vi "refMgr_Example4.vi"() -> ()   [LabVIEW 2017]
uses:
  RefManager/Typedef/RefMgr-Logic-State.ctl
  RefManager/Typedef/RefMgr-StateChangeType.ctl
  40be52e9-3771-4604-be95-a9dd39ca470b.vi
  <userlib>/_NEVSTOP/TagDB/_Support/DataAccess/data-Write.vi
  <userlib>/_NEVSTOP/TagDB/_Support/DataAccess/_NameCacher.vi
  <userlib>/_NEVSTOP/TagDB/_Support/DataAccess/_datatypeChecker.vi
  <userlib>/_NEVSTOP/TagDB/_Support/DataAccess/TagDB Ref to DVR.vi
  <vilib>/Utility/Data Type/Get Type Information.vi
  <vilib>/Utility/error.llb/Trim Whitespace.vi
  <userlib>/_NEVSTOP/TagDB/_Support/Error/_[error50000]Invalid DB REF.vi
  RefManager/TagDB RefManager.lvlib
  <userlib>/_NEVSTOP/TagDB/TagDB.lvlib
panel:
  in  "StateValue":i16
  in  "stop":bool
  in  "Boolean 6":bool
  in  "Boolean 5":bool
  in  "Boolean 4":bool
  in  "Boolean 3":bool
  in  "Boolean 2":bool
  in  "Boolean 1":bool
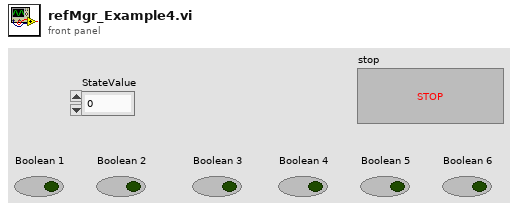
[diagram p1: front panel]
types:
  T1 = typedef "TagDB RefManager.lvlib/RefMgr-Logic-State.ctl" = cluster{"StateName":string, "StateValue":i32, "Type":T2, "Calcs":cluster{"Tag":string, "Exp":string}[]}
  T2 = typedef "TagDB RefManager.lvlib/RefMgr-StateChangeType.ctl" = enum16{"0 - 进入", "1 - 等于", "2 - 退出"}
  T3 = typedef "TagDB.lvlib/TagDB.ctl" = refnum<k1>
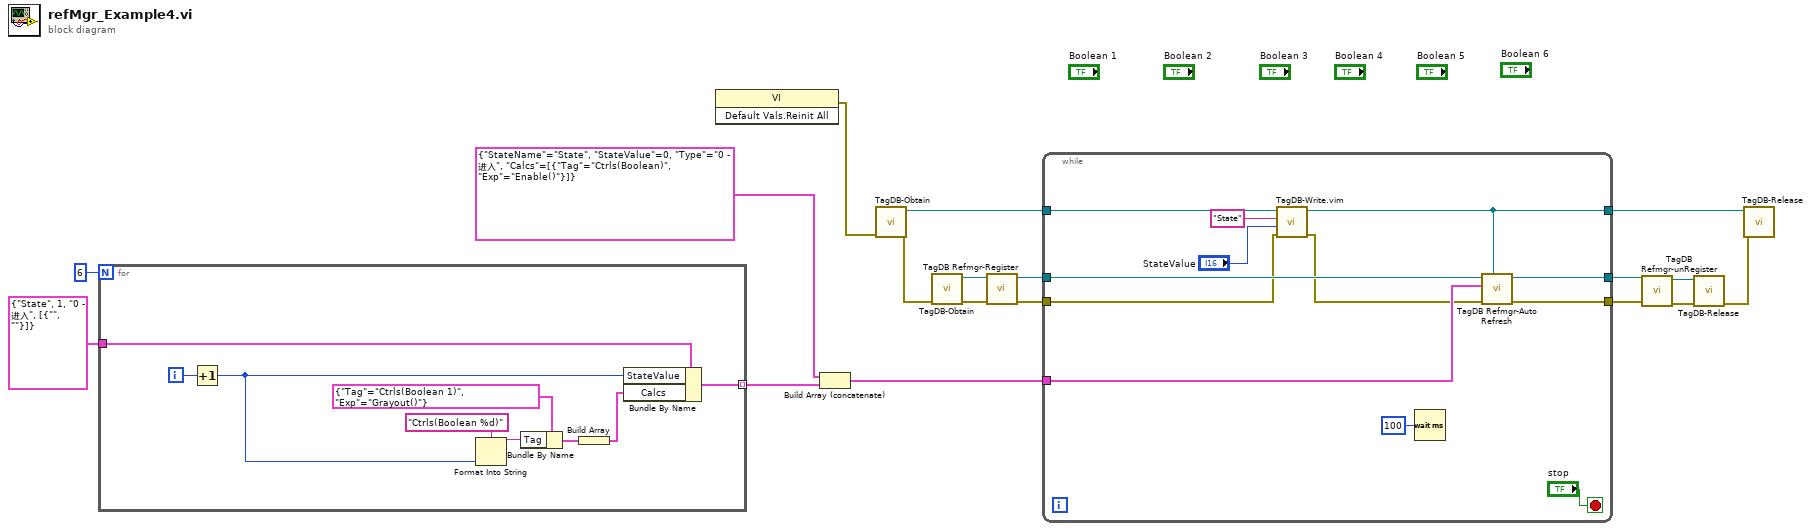
[diagram p0: block diagram]
diagram:
  n1 = for {
    N: 6 -> [_]
    tunnel: T1 {"StateName"="State", "StateValue"=1, "Type"=enum."0 - 进入", "Calcs"=[{"Tag"="", "Exp"=""}]} ("Cluster") -> [w27]
    tunnel: [w20] -> w10 mode=indexing
    i -> [w25]
    n2 = Increment(x=w25) -> (x+1=w19:i32)
    n3 = Format Into String(format string="Ctrls(Boolean %d)" ("Tag"), w19) -> (resulting string=w23:string)  [unwired: 2 in, 1 out]
    n4 = Bundle By Name(cluster=cluster{"Tag":string, "Exp":string} {"Tag"="Ctrls(Boolean 1)", "Exp"="Grayout()"} ("Cluster"), "Tag"=w23) -> (w22:cluster{"Tag":string, "Exp":string})
    n5 = Build Array(w22) -> (w21:cluster{"Tag":string, "Exp":string}[])
    n6 = Bundle By Name(cluster=w27, "StateValue"=w19, "Calcs"=w21) -> (w20:T1)
  }
  n7 = invoke class="VI" method="Default Vals.Reinit All"() -> (error out=w1:errorcluster)  [unwired: 3 in, 2 out]
  n8 = Build Array (concatenate)(T1 {"StateName"="State", "StateValue"=0, "Type"=enum."0 - 进入", "Calcs"=[{"Tag"="Ctrls(Boolean)", "Exp"="Enable()"}]} ("Cluster"), w10) -> (w9:T1[])
  n9 = call <userlib>:"TagDB-Obtain.vi"("error in (no error)"=w1) -> ("error out"=w14:errorcluster, "TagDB"=w13:T3)  [unwired: 4 in, 1 out]
  n10 = call <userlib>:"TagDB-Obtain.vi"("error in (no error)"=w14) -> ("error out"=w17:errorcluster, "TagDB"=w18:T3)  [unwired: 4 in, 1 out]
  n11 = call "TagDB Refmgr-Register.vi"("error in (no error)"=w17, "TagDB in"=w18) -> ("error out"=w15:errorcluster, "TagDB out"=w16:T3)  [unwired: 7 in, 1 out]
  n12 = while {
    tunnel: w16 -> [w39]
    tunnel: w15 -> [w29]
    tunnel: w13 -> [w33]
    tunnel: w9 -> [w38]
    tunnel: [w35] -> w5
    tunnel: [w34] -> w4
    tunnel: [w32] -> w3
    stop <- "stop" stop-if-true
    n13 = call "TagDB-Write.vim"("error in (no error)"=w29, "Value"="StateValue", "name"="State", "TagDB"=w33) -> ("error out"=w28:errorcluster, "TagDB(dup)"=w32:T3)  [unwired: 5 in, 1 out]
    n14 = Wait (ms)(milliseconds to wait=u32 100) -> ()  [unwired: 1 out]
    n15 = call "TagDB Refmgr-Auto Refresh.vi"("DataDB"=w32, "error in (no error)"=w28, "Rules"=w38, "DB Ref"=w39) -> ("error out"=w34:errorcluster, "DB Ref (dup)"=w35:T3)  [unwired: 6 in]
  }
  n16 = call "TagDB Refmgr-unRegister.vi"("error in (no error)"=w4, "TagDB in"=w5) -> ("error out"=w7:errorcluster, "TagDB out"=w6:T3)  [unwired: 8 in]
  n17 = call <userlib>:"TagDB-Release.vi"("error in (no error)"=w7, "TagDB"=w6) -> ("error out"=w2:errorcluster)  [unwired: 9 in]
  n18 = call <userlib>:"TagDB-Release.vi"("error in (no error)"=w2, "TagDB"=w3) -> ()  [unwired: 9 in, 1 out]
